vi "New Log.vi"(6 "Path (optional)":path, 8 "error in (no error)":errorcluster, 9 "Specific Error Code":i32, 10 "Name":string) -> (0 "error out":errorcluster, 3 "Log out":refnum<class "Log.lvclass">)   [LabVIEW 2026, in "TALOS.lvlib" / "Classes.lvlib" / "Log.lvclass"]
doc: "This VI creates a new log file to be used for a specific purpouse (for general purpouse, use the common System one). The path is automatically generated, unless specified in input.\nThe file generated is automatically rotated every 7 days."
uses:
  Log.lvclass
  Ancestor/Ancestor/Ancestor.lvclass/Ancestor.ctl
  Log.lvclass/Log.ctl
  FGV/Error Memory/Get Error Description.vi
  Support VIs/Get PC name.vi
  Ancestor/Ancestor/Read ID.vi
  Support VIs/Get Class Name.vi
  <vilib>/Utility/error.llb/Clear Errors.vi
  FGV/Error Memory/Error Memory Core.vi
  <vilib>/AdvancedString/Delimited String to 1D String Array.vi
  <vilib>/AdvancedString/Delimited String to 1D String Array (string).vi
  Support VIs/Circus Root Path.vi
  FGV/Error Memory/Error Crt Lvl checker.vi
  FGV/Error Memory/Error Memory Core.vi/40c8088d-b597-4017-91af-faa98e00292e.vi
  FGV/Error Memory/Error Memory Core.vi/d4a3ab98-063c-4e44-b43d-fbdcfe6c2be2.vi
  Support VIs/Global Memory.vi
  <vilib>/Utility/LVClass/Get LV Class Name.vi
  Support VIs/Is in Packed Library.vi
  Support VIs/TALOS Root path.vi
  Support VIs/Read CSV worksheet.vi
  Support VIs/Global Constants.vi
  <vilib>/Utility/error.llb/General Error Handler.vi
  <vilib>/Utility/config.llb/Open Config Data.vi
  <vilib>/Utility/config.llb/Get Section Names.vi
  <vilib>/Utility/config.llb/Get Key Names.vi
  <vilib>/Utility/config.llb/Read Key.vi
  <vilib>/Utility/config.llb/Read Key (String).vi
  <vilib>/Utility/config.llb/Close Config Data.vi
  <vilib>/Utility/error.llb/Search and Replace Pattern.vi
  <vilib>/Utility/error.llb/Search and Replace Pattern (string).vi
  Ancestor/Ancestor/Ancestor.lvclass
  <vilib>/Comparison/Equal/Equal Functor/Equal Functor.lvclass
  TALOS.lvlib
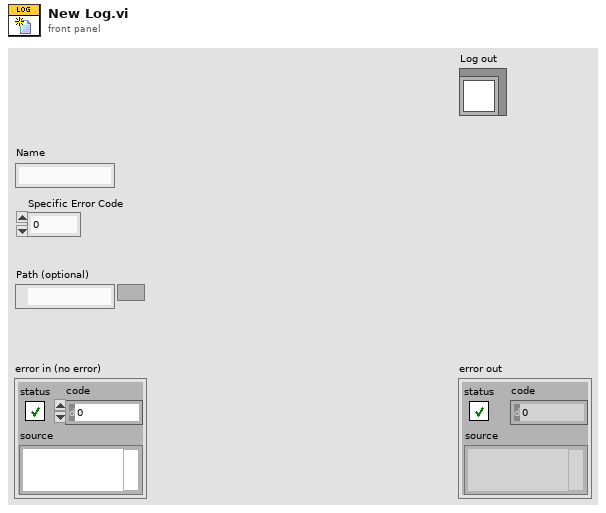
[diagram p1: front panel]
types:
  T1 = enum16{"open", "replace", "create", "open or create", "replace or create", "replace or create with confirmation"}
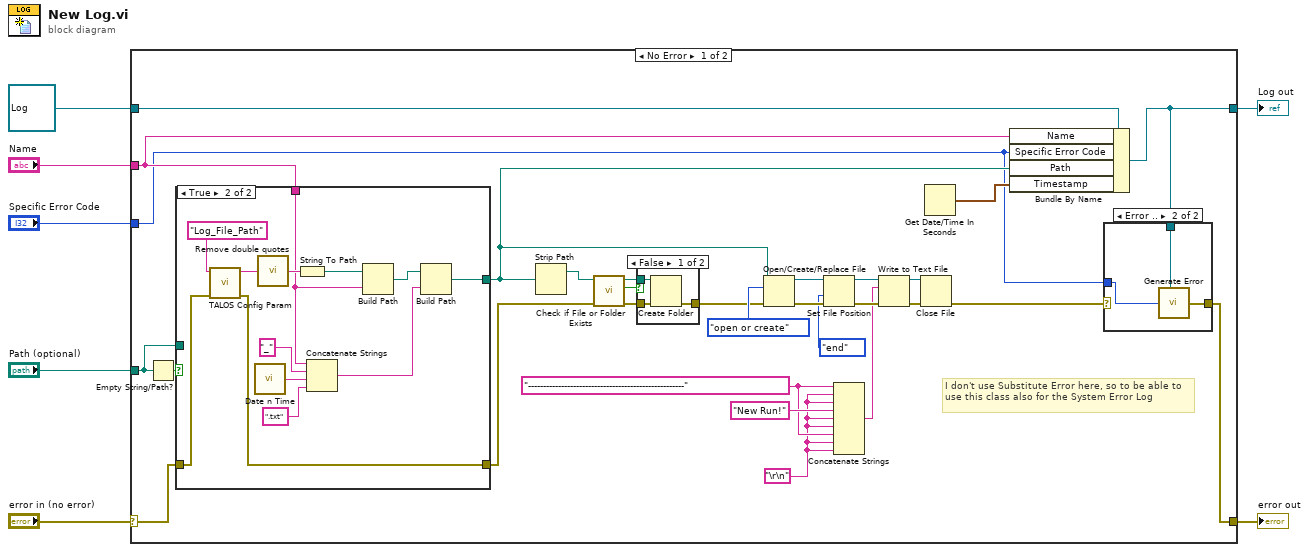
[diagram p0: block diagram]
diagram:
  n1 = case shown="No Error" "error in (no error)" {
    selector: "error in (no error)" -> [w32 w61]
    tunnel: [w8 w61] -> w6
    tunnel: [w9 w60] -> w5
    tunnel: refnum<class "Log.lvclass"> refnum ("Log in") -> [w36 w60]
    tunnel: "Path (optional)" -> [w34 _]
    tunnel: "Name" -> [w33 _]
    tunnel: "Specific Error Code" -> [w10 _]
    frame No Error {
      w22 = "----------------------------------------------------"
      w21 = "\r\n"
      # "I don't use Substitute Error here, so to be able to use this class also for the System Error Log"
      n2 = Empty String/Path?(string/path=w34) -> (empty?=w35:bool)
      n3 = case shown="True" w35 {
        tunnel: w34 -> [w45 _]
        tunnel: w33 -> [_ w48]
        tunnel: w32 -> [w46 w53]
        tunnel: [w45 w52] -> w14
        tunnel: [w46 w51] -> w13
        frame False {
        }
        frame True {
          n4 = call "TALOS Config Param.vi"("error in (no error)"=w53, "Parameter Name"="Log_File_Path") -> ("error out"=w51:errorcluster, "Output"=w55:string)  [unwired: 8 in]
          n5 = call "Date n Time.vi"() -> ("Date & Time"=w58:string)  [unwired: 5 in]
          n6 = call "Remove double quotes.vi"("Input string"=w55) -> ("Output string"=w54:string)  [unwired: 4 in]
          n7 = String To Path(string=w54) -> (path=w50:path)
          n8 = Concatenate Strings(w48, "_" ("string"), w58, ".txt" ("string")) -> (w57:string)
          n9 = Build Path(base path=w50, name or relative path=w48) -> (appended path=w49:path)
          n10 = Build Path(base path=w49, name or relative path=w57) -> (appended path=w52:path)
        }
      }
      n11 = Strip Path(path=w14) -> (stripped path=w16:path)  [unwired: 1 out]
      n12 = call <vilib>:"Check if File or Folder Exists.vi"("error in (no error)"=w13, "path"=w16) -> ("error out"=w18:errorcluster, "file or folder exists?"=w19:bool, "dup path"=w17:path)  [unwired: 7 in]
      n13 = case shown="False" w19 {
        tunnel: w17 -> [w43 _]
        tunnel: w18 -> [w42 w44]
        tunnel: [w41 w44] -> w15
        frame False {
          n14 = Create Folder(path (use dialog)=w43, error in=w42) -> (error out=w41:errorcluster)  [unwired: 1 in, 2 out]
        }
        frame True {
        }
      }
      n15 = Open/Create/Replace File(file path (use dialog)=w14, error in=w15, operation (0:open)=T1."open or create") -> (refnum out=w30:refnum<file>, error out=w29:errorcluster)  [unwired: 3 in, 1 out]
      n16 = Set File Position(refnum=w30, from (0:start)=enum16{"start", "end", "current"}."end", error in=w29) -> (refnum out=w25:refnum<file>, error out=w27:errorcluster)  [unwired: 1 in]
      n17 = Concatenate Strings(w22, w21, w21, "New Run!", w21, w21, w22, w21, w21) -> (w20:string)
      n18 = Write to Text File(file (use dialog)=w25, text=w20, error in=w27) -> (refnum out=w24:refnum<file>, error out=w26:errorcluster)  [unwired: 1 in, 1 out]
      n19 = Close File(refnum=w24, error in=w26) -> (error out=w11:errorcluster)  [unwired: 1 out]
      n20 = Get Date/Time In Seconds() -> (seconds since 1Jan1904=w12:timestamp)
      n21 = Bundle By Name(cluster=w36, "Name"=w33, "Specific Error Code"=w10, "Path"=w14, "Timestamp"=w12) -> (w9:refnum<class "Log.lvclass">)
      n22 = case shown="Error .." w11 {
        selector: w11 -> [w37 _]
        tunnel: [w37 w40] -> w8
        tunnel: w10 -> [_ w39]
        tunnel: w9 -> [_ w38]
        frame No Error {
        }
        frame Error {
          n23 = call "Generate Error.vi"("Class"=w38, "Error Code"=w39) -> ("error out"=w40:errorcluster)  [unwired: 5 in]
        }
      }
    }
    frame Error {
    }
  }
  "error out" <- w6
  "Log out" <- w5
